vi "practica2_ejercicio4.vi"   [LabVIEW 2011]
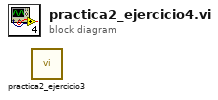
[diagram p0: block diagram]
diagram:
  n1 = call "practica2_ejercicio3.vi"() -> ()  [unwired: 3 in, 5 out]
